vi "Forebrain old.vi"() -> ()   [LabVIEW 2011]
uses:
  Behaviour.ctl
  MDF.ctl
  Position.ctl
panel:
  out "Behavior":T1
  in  "Threshold 4":dbl
  in  "Threshold 3":dbl
  in  "Threshold 2":dbl
  in  "Threshold":dbl
  in  "Current State":i16
  out "Draw?":bool
  in  "stop":bool
  out "MDF":T2[](array[typedef])
  in  "Tab Control":enum32{"Mission Planning", "Auto-Mode"}(tab)
  in  "Behaviour":T1
  out "No. of Waypoints":i16
  out "Waypoint Index":i16
  in  "Speed":dbl(slide) scale=0.0..10.0
  out "Mission Definition":picture
  in  "path to PNG file":path
  out "Boat":T3
  out "Buoy2":T3
  out "Buoy1":T3
  out "Dock":T3
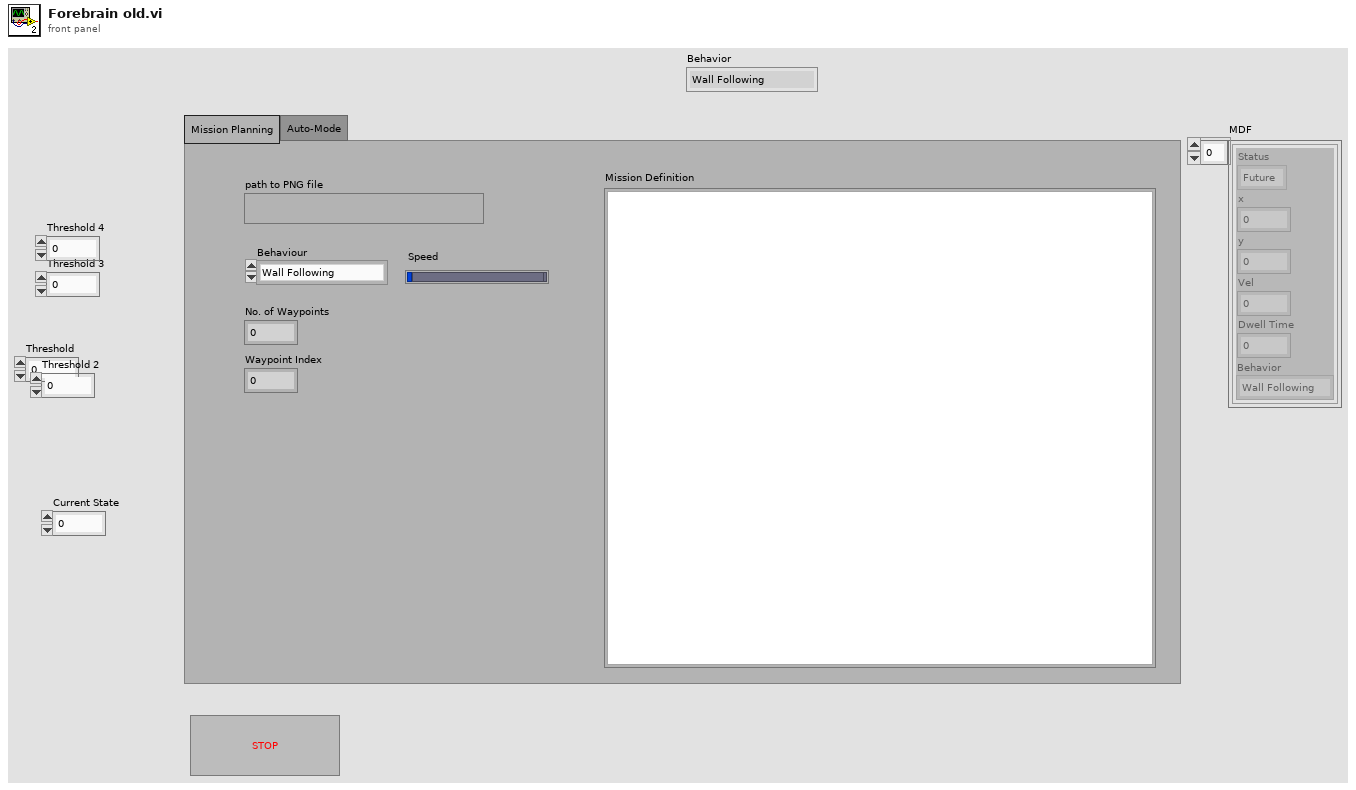
[diagram p1: front panel]
types:
  T1 = typedef "Behaviour.ctl" = enum16{"Wall Following", "Open Transit", "Find Barge", "Home"}
  T2 = typedef "MDF.ctl" = cluster{"Status":enum16{"Past", "Current", "Future"}, "x":dbl, "y":dbl, "Vel":dbl, "Dwell Time":dbl, "Behavior":T1}
  T3 = typedef "Position.ctl" = cluster{"X":sgl, "Y":sgl}
  T4 = cluster{"Status":enum16{"Past", "Current", "Future"}, "x":dbl, "y":dbl, "Vel":dbl, "Dwell Time":dbl, "Behavior":T1}[]
  T5 = typedef "imagedata.ctl" = cluster{"image type":i32, "image depth":i32, "image":u8[], "mask":u8[], "colors":u32[], "Rectangle":cluster{"left":i16, "top":i16, "right":i16, "bottom":i16}}
  T6 = cluster{"Status":enum16{"Past", "Current", "Future"}, "x":dbl, "y":dbl, "Vel":dbl, "Dwell Time":dbl, "Behaviour":T1}
  T7 = cluster{"Width":u16, "Style":enum32{"Solid", "Dash", "Dot", "DashDot", "DashDotDot"}}
  T8 = typedef "LVMouseTypeDef.ctl" = cluster{"Mouse Position":cluster{"X":i32, "Y":i32}, "Mouse Modifiers":cluster{"Button Down":bool, "Shift Mod":bool, "Menu Mod":bool, "Option Mod":bool}}
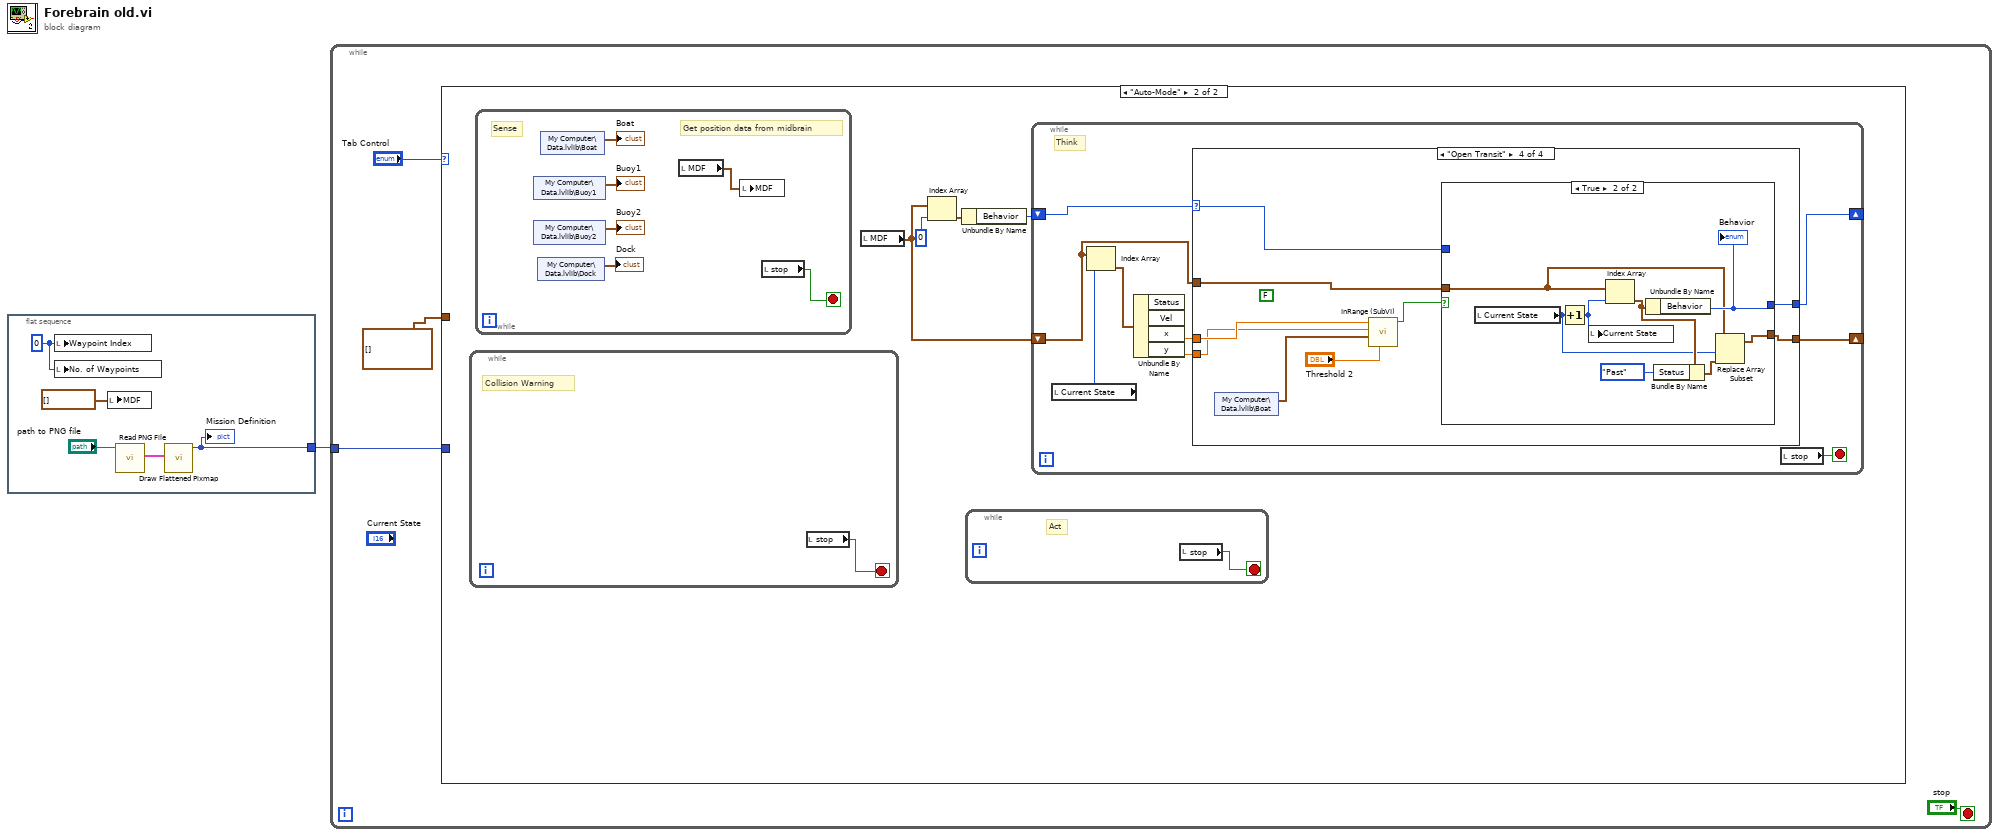
[diagram p0: block diagram]
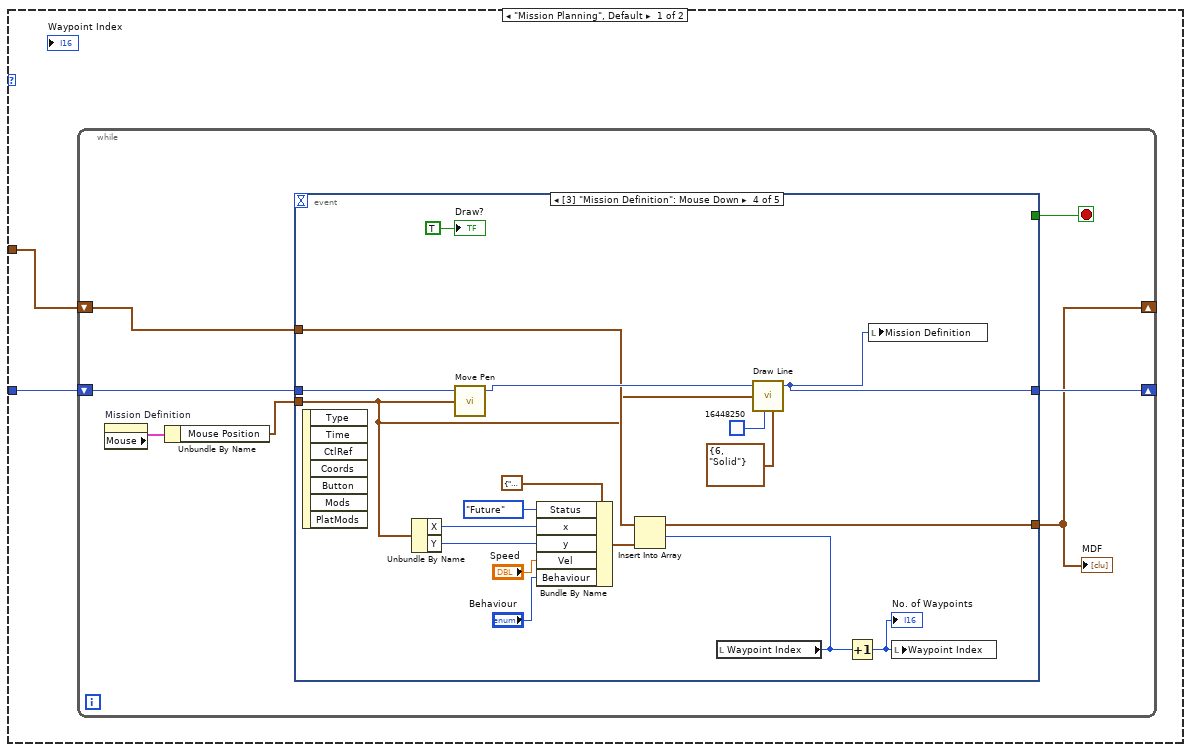
[diagram p2: hidden frame]
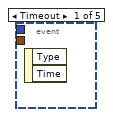
[diagram p3: hidden frame]
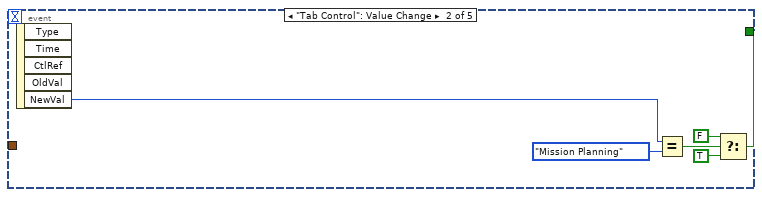
[diagram p4: hidden frame]
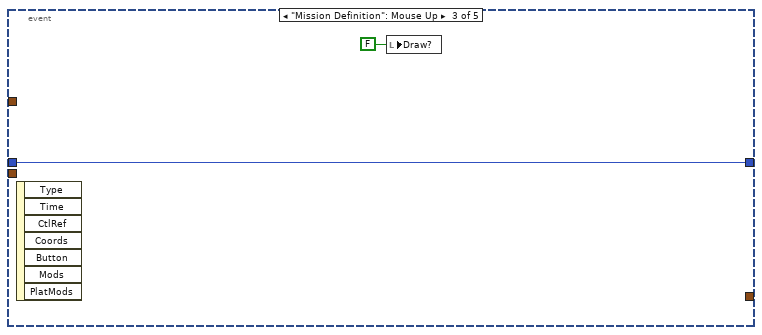
[diagram p5: hidden frame]
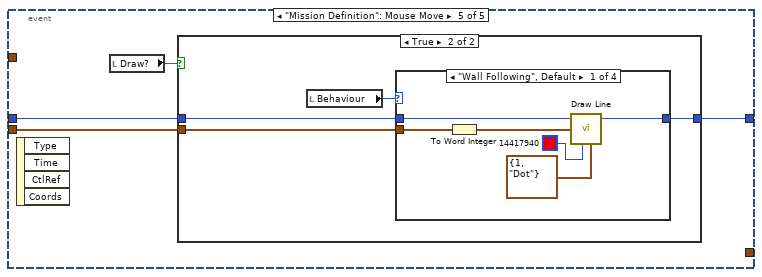
[diagram p6: hidden frame]
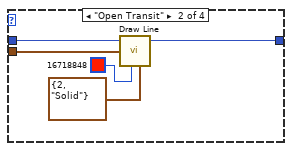
[diagram p8: hidden frame]
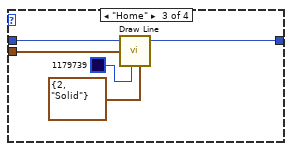
[diagram p9: hidden frame]
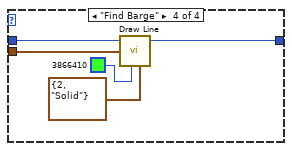
[diagram p10: hidden frame]
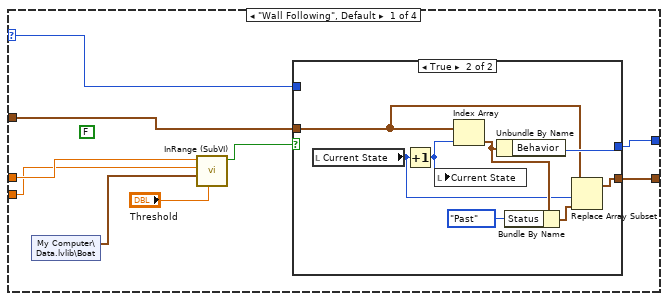
[diagram p11: hidden frame]
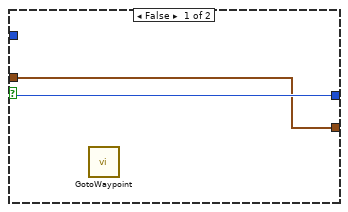
[diagram p12: hidden frame]
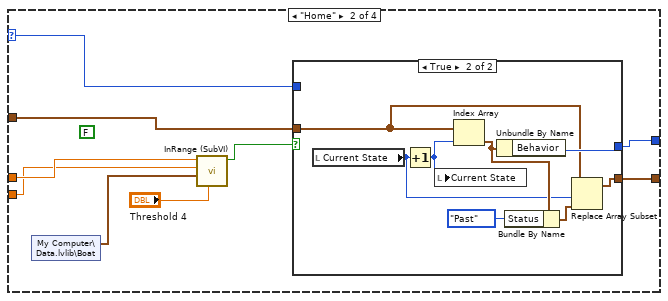
[diagram p13: hidden frame]
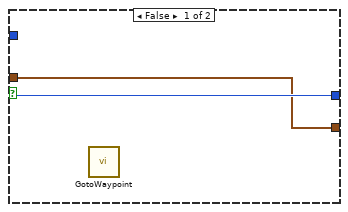
[diagram p14: hidden frame]
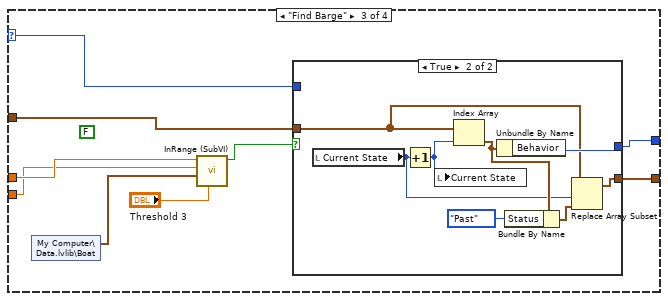
[diagram p15: hidden frame]
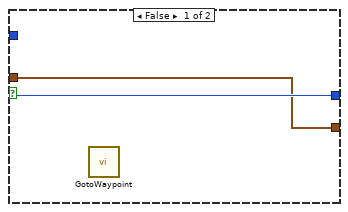
[diagram p16: hidden frame]
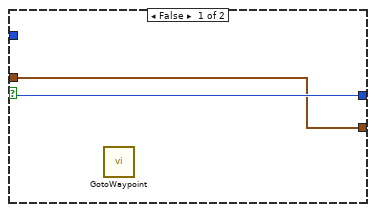
[diagram p17: hidden frame]
diagram:
  n1 = flat-sequence {
    tunnel: [w4] -> w1
    frame #0 {
      w3 = i16 0 ("No. of Waypoints")
      n2 = local write "Waypoint Index"(w3) -> ()
      n3 = local write "No. of Waypoints"(w3) -> ()
      n4 = local write "MDF"(T4 [] ("MDF")) -> ()
      n5 = call <vilib>:"Read PNG File.vi"("path to PNG file"="path to PNG file") -> ("image data"=w6:T5)  [unwired: 8 in, 2 out]
      n6 = call <vilib>:"Draw Flattened Pixmap.vi"("image data"=w6) -> ("new picture"=w4:picture)  [unwired: 8 in]
      "Mission Definition" <- w4
    }
  }
  n7 = while {
    tunnel: w1 -> [w8]
    stop <- "stop" stop-if-true
    n8 = case shown="\"Auto-Mode\"" "Tab Control" {
      tunnel: w8 -> [w12 _]
      tunnel: T2[] [] ("MDF") -> [w11 _]
      frame "Mission Planning", Default {
        n9 = while {
          shift-right: [w15] -> _
          shift-left: w11 -> [w19]
          shift-right: [w16] -> _
          shift-left: w12 -> [w17]
          stop <- w18 stop-if-true
          n10 = property on="Mission Definition" class="Pict"() -> ("Mouse"=w14:T8)  [unwired: 2 in, 2 out]
          n11 = Unbundle By Name(w14) -> ("Mouse Position"=w13:cluster{"X":i32, "Y":i32})
          n12 = event shown="[3] \"Mission Definition\": Mouse Down" {
            selector: _ -> [_ _ _ _ _]
            dyn-events: _ -> [_ _ _ _ _]
            timeout: _ -> [_ _ _ _ _]
            tunnel: w19 -> [_ _ _ w42 _]
            tunnel: [_ _ _ w35 _] -> w15
            tunnel: [_ w20 _ _ _] -> w18
            tunnel: w17 -> [_ _ w26 w34 w47]
            tunnel: [_ _ w26 w28 w46] -> w16
            tunnel: w13 -> [_ _ _ w29 w48]
            event Timeout {
              n13 = event-data() -> ()  [unwired: 1 in, 2 out]
            }
            event "Tab Control": Value Change {
              n14 = event-data() -> ("NewVal"=w25:enum32{"Mission Planning", "Auto-Mode"})  [unwired: 1 in, 4 out]
              n15 = Equal?(x=w25, y=enum32{"Mission Planning", "Auto-Mode"}."Mission Planning") -> (x = y?=w23:bool)
              n16 = Select(t=FALSE, s=w23, f=TRUE) -> (s? t:f=w20:bool)
            }
            event "Mission Definition": Mouse Up {
              n17 = event-data() -> ()  [unwired: 1 in, 7 out]
              n18 = local write "Draw?"(FALSE ("Draw?")) -> ()
            }
            event "Mission Definition": Mouse Down {
              n19 = event-data() -> ()  [unwired: 1 in, 7 out]
              n20 = Unbundle By Name(w29) -> ("X"=w41:i32, "Y"=w40:i32)
              n21 = call <vilib>:"Move Pen.vi"("new position"=w29, "picture"=w34) -> ("new picture"=w45:picture)  [unwired: 3 in]
              n22 = Bundle By Name(cluster=T6 {"Status"=enum."Future", "x"=0.0, "y"=0.0, "Vel"=0.0, "Dwell Time"=0.0, "Behaviour"=enum."Wall Following"} ("MissionDefinitionFile"), "Status"=enum16{"Past", "Current", "Future"}."Future", "x"=w41, "y"=w40, "Vel"="Speed", "Behaviour"="Behaviour") -> (w31:T6)
              n23 = local read "Waypoint Index"() -> (w39:i16)
              n24 = Insert Into Array(array=w42, index=w39, new element=w31) -> (w35:T2[])
              n25 = call <vilib>:"Draw Line.vi"("picture"=w45, "end point"=w29, "color(black)"=u32 16448250, "pen"=T7 {"Width"=6, "Style"=enum."Solid"}) -> ("new picture"=w28:picture)  [unwired: 5 in]
              n26 = Increment(x=w39) -> (x+1=w38:i16)
              "No. of Waypoints" <- w38
              n27 = local write "Mission Definition"(w28) -> ()
              n28 = local write "Waypoint Index"(w38) -> ()
              "Draw?" <- TRUE ("Draw?")
            }
            event "Mission Definition": Mouse Move {
              n29 = event-data() -> ()  [unwired: 1 in, 4 out]
              n30 = local read "Draw?"() -> (w49:bool)
              n31 = case shown="True" w49 {
                tunnel: w48 -> [_ w54]
                tunnel: w47 -> [w50 w53]
                tunnel: [w50 w52] -> w46
                frame False {
                }
                frame True {
                  n32 = local read "Behaviour"() -> (w51:T1)
                  n33 = case shown="\"Wall Following\", Default" w51 {
                    tunnel: w54 -> [w56 w65 w70 w75]
                    tunnel: w53 -> [w60 w62 w67 w72]
                    tunnel: [w57 w61 w66 w71] -> w52
                    frame "Wall Following", Default {
                      n34 = To Word Integer(number=w56) -> (16bit integer=w55:cluster{"X":i16, "Y":i16})
                      n35 = call <vilib>:"Draw Line.vi"("picture"=w60, "end point"=w55, "color(black)"=u32 14417940, "pen"=T7 {"Width"=1, "Style"=enum."Dot"}) -> ("new picture"=w57:picture)  [unwired: 5 in]
                    }
                    frame "Open Transit" {
                      n36 = call <vilib>:"Draw Line.vi"("picture"=w62, "end point"=w65, "color(black)"=u32 16718848, "pen"=T7 {"Width"=2, "Style"=enum."Solid"}) -> ("new picture"=w61:picture)  [unwired: 5 in]
                    }
                    frame "Home" {
                      n37 = call <vilib>:"Draw Line.vi"("picture"=w67, "end point"=w70, "color(black)"=u32 1179739, "pen"=T7 {"Width"=2, "Style"=enum."Solid"}) -> ("new picture"=w66:picture)  [unwired: 5 in]
                    }
                    frame "Find Barge" {
                      n38 = call <vilib>:"Draw Line.vi"("picture"=w72, "end point"=w75, "color(black)"=u32 3866410, "pen"=T7 {"Width"=2, "Style"=enum."Solid"}) -> ("new picture"=w71:picture)  [unwired: 5 in]
                    }
                  }
                }
              }
            }
          }
          "MDF" <- w15
        }
      }
      frame "Auto-Mode" {
        n39 = while {
          stop <- w80 stop-if-true
          # "Collision Warning"
          n40 = local read "stop"() -> (w80:bool)
        }
        n41 = while {
          stop <- w168 stop-if-true
          # "Get position data from midbrain"
          # "Sense"
          n42 = shared-variable "My Computer\\Data.lvlib\\Buoy1"() -> (→"Buoy1":T3)  [unwired: 1 in, 1 out]
          n43 = shared-variable "My Computer\\Data.lvlib\\Buoy2"() -> (→"Buoy2":T3)  [unwired: 1 in, 1 out]
          n44 = shared-variable "My Computer\\Data.lvlib\\Dock"() -> (→"Dock":T3)  [unwired: 1 in, 1 out]
          n45 = shared-variable "My Computer\\Data.lvlib\\Boat"() -> (→"Boat":T3)  [unwired: 1 in, 1 out]
          n46 = local read "MDF"() -> (w167:T2[])
          n47 = local write "MDF"(w167) -> ()
          n48 = local read "stop"() -> (w168:bool)
        }
        n49 = local read "MDF"() -> (w76:T2[])
        n50 = Index Array(array=w76, index=0) -> (element=w78:T2)
        n51 = Unbundle By Name(w78) -> ("Behavior"=w77:T1)
        n52 = while {
          stop <- w81 stop-if-true
          # "Act"
          n53 = local read "stop"() -> (w81:bool)
        }
        n54 = while {
          shift-right: [w89] -> _
          shift-left: w77 -> [w88]
          shift-right: [w82] -> _
          shift-left: w76 -> [w87]
          stop <- w90 stop-if-true
          # "Think"
          n55 = local read "Current State"() -> (w86:i16)
          n56 = Index Array(array=w87, index=w86) -> (element=w85:T2)
          n57 = Unbundle By Name(w85) -> ("x"=w84:dbl, "y"=w83:dbl)  [unwired: 2 out]
          n58 = case shown="\"Open Transit\"" w88 {
            selector: w88 -> [w97 w116 w135 w154]
            tunnel: [w99 w118 w137 w156] -> w89
            tunnel: w87 -> [w98 w117 w136 w155]
            tunnel: w84 -> [w95 w114 w133 w152]
            tunnel: w83 -> [w94 w113 w132 w151]
            tunnel: [w91 w110 w129 w148] -> w82
            frame "Wall Following", Default {
              (unwired) FALSE
              n59 = shared-variable "My Computer\\Data.lvlib\\Boat"() -> (w96:T3)  [unwired: 1 in, 1 out]
              n60 = call "InRange (SubVI).vi"("Threshold"="Threshold", "Boat Position"=w96, "y"=w94, "x"=w95) -> ("In Range?"=w93:bool)  [unwired: 7 in]
              n61 = case shown="True" w93 {
                tunnel: [w101 w109] -> w99
                tunnel: w98 -> [w100 w105]
                tunnel: w97 -> [w101 _]
                tunnel: [w100 w102] -> w91
                frame False {
                  n62 = call "GotoWaypoint.vi"() -> ()  [unwired: 6 in, 6 out]
                }
                frame True {
                  n63 = local read "Current State"() -> (w103:i16)
                  n64 = Increment(x=w103) -> (x+1=w108:i16)
                  n65 = local write "Current State"(w108) -> ()
                  n66 = Index Array(array=w105, index=w108) -> (element=w107:T2)
                  n67 = Unbundle By Name(w107) -> ("Behavior"=w109:T1)
                  n68 = Bundle By Name(cluster=w107, "Status"=enum16{"Past", "Current", "Future"}."Past") -> (w104:T2)
                  n69 = Replace Array Subset(array=w105, new element=w104, index=w103) -> (w102:T2[])
                }
              }
            }
            frame "Home" {
              (unwired) FALSE
              n70 = shared-variable "My Computer\\Data.lvlib\\Boat"() -> (w115:T3)  [unwired: 1 in, 1 out]
              n71 = call "InRange (SubVI).vi"("Threshold"="Threshold 4", "Boat Position"=w115, "y"=w113, "x"=w114) -> ("In Range?"=w112:bool)  [unwired: 7 in]
              n72 = case shown="True" w112 {
                tunnel: [w120 w128] -> w118
                tunnel: w117 -> [w119 w124]
                tunnel: w116 -> [w120 _]
                tunnel: [w119 w121] -> w110
                frame False {
                  n73 = call "GotoWaypoint.vi"() -> ()  [unwired: 6 in, 6 out]
                }
                frame True {
                  n74 = local read "Current State"() -> (w122:i16)
                  n75 = Increment(x=w122) -> (x+1=w127:i16)
                  n76 = local write "Current State"(w127) -> ()
                  n77 = Index Array(array=w124, index=w127) -> (element=w126:T2)
                  n78 = Unbundle By Name(w126) -> ("Behavior"=w128:T1)
                  n79 = Bundle By Name(cluster=w126, "Status"=enum16{"Past", "Current", "Future"}."Past") -> (w123:T2)
                  n80 = Replace Array Subset(array=w124, new element=w123, index=w122) -> (w121:T2[])
                }
              }
            }
            frame "Find Barge" {
              (unwired) FALSE
              n81 = shared-variable "My Computer\\Data.lvlib\\Boat"() -> (w134:T3)  [unwired: 1 in, 1 out]
              n82 = call "InRange (SubVI).vi"("Threshold"="Threshold 3", "Boat Position"=w134, "y"=w132, "x"=w133) -> ("In Range?"=w131:bool)  [unwired: 7 in]
              n83 = case shown="True" w131 {
                tunnel: [w139 w147] -> w137
                tunnel: w136 -> [w138 w143]
                tunnel: w135 -> [w139 _]
                tunnel: [w138 w140] -> w129
                frame False {
                  n84 = call "GotoWaypoint.vi"() -> ()  [unwired: 6 in, 6 out]
                }
                frame True {
                  n85 = local read "Current State"() -> (w141:i16)
                  n86 = Increment(x=w141) -> (x+1=w146:i16)
                  n87 = local write "Current State"(w146) -> ()
                  n88 = Index Array(array=w143, index=w146) -> (element=w145:T2)
                  n89 = Unbundle By Name(w145) -> ("Behavior"=w147:T1)
                  n90 = Bundle By Name(cluster=w145, "Status"=enum16{"Past", "Current", "Future"}."Past") -> (w142:T2)
                  n91 = Replace Array Subset(array=w143, new element=w142, index=w141) -> (w140:T2[])
                }
              }
            }
            frame "Open Transit" {
              (unwired) FALSE
              n92 = shared-variable "My Computer\\Data.lvlib\\Boat"() -> (w153:T3)  [unwired: 1 in, 1 out]
              n93 = call "InRange (SubVI).vi"("Threshold"="Threshold 2", "Boat Position"=w153, "y"=w151, "x"=w152) -> ("In Range?"=w150:bool)  [unwired: 7 in]
              n94 = case shown="True" w150 {
                tunnel: [w158 w166] -> w156
                tunnel: w155 -> [w157 w162]
                tunnel: w154 -> [w158 _]
                tunnel: [w157 w159] -> w148
                frame False {
                  n95 = call "GotoWaypoint.vi"() -> ()  [unwired: 6 in, 6 out]
                }
                frame True {
                  n96 = local read "Current State"() -> (w160:i16)
                  n97 = Increment(x=w160) -> (x+1=w165:i16)
                  n98 = local write "Current State"(w165) -> ()
                  n99 = Index Array(array=w162, index=w165) -> (element=w164:T2)
                  n100 = Unbundle By Name(w164) -> ("Behavior"=w166:T1)
                  "Behavior" <- w166
                  n101 = Bundle By Name(cluster=w164, "Status"=enum16{"Past", "Current", "Future"}."Past") -> (w161:T2)
                  n102 = Replace Array Subset(array=w162, new element=w161, index=w160) -> (w159:T2[])
                }
              }
            }
          }
          n103 = local read "stop"() -> (w90:bool)
        }
      }
    }
  }
